vi "write_lockin_FP_DSC.vi"(8 "error in (no error)":errorcluster, 11 "front panel":T1 {"AI Configuration"."AI.Coupling" items=["AC"=10045, "DC"=10050, "GND"=10066]; "Channels: AO"."AO f (Hz)" min=0.001 max=10000.0; "Channels: AO"."AO DC (V)" format="%.3p"; "Channels: AO"."AO Amp (V)" format="%.3p"; "Channels: Lockin"."REF phi (°)" format="%#_3g"}) -> (0 "error out":errorcluster)   [LabVIEW 2016, in "Instrument.Lockin.lvclass"]
uses:
  Instrument.Lockin.lvclass
  Typedefs/Front Panel Cluster.ctl
  Typedefs/AO.config(UI)-array.ctl
  Typedefs/AO.config(UI)-cluster.ctl
  Typedefs/446xAO-enum.ctl
  Typedefs/AI.config(UI)-array.ctl
  Typedefs/AI.config(UI)-cluster.ctl
  Typedefs/AI.coupling-enum.ctl
  Typedefs/446xAI-enum.ctl
  Typedefs/AO-cluster.ctl
  Typedefs/AO_Amp-array.ctl
  Typedefs/AO_DC-array.ctl
  Typedefs/AO_f-array.ctl
  Typedefs/AO_phi-array.ctl
  Typedefs/Function-array.ctl
  Typedefs/Function-enum.ctl
  Typedefs/REF-cluster.ctl
  Typedefs/REF_f-array.ctl
  Typedefs/REF_phi-array.ctl
  Typedefs/DAQType-enum.ctl
  Typedefs/AmplifierType-enum.ctl
  Typedefs/Cal Info - Cluster.ctl
  <vilib>/Utility/sysdir.llb/System Directory Type.ctl
  <vilib>/addons/_JKI.lib/Serialization/JSON/JKI JSON Serialization.lvlib
panel:
  # "1"
  # "2"
  # "3"
  # "4"
  # "5"
  # "6"
  # "7"
  # "8"
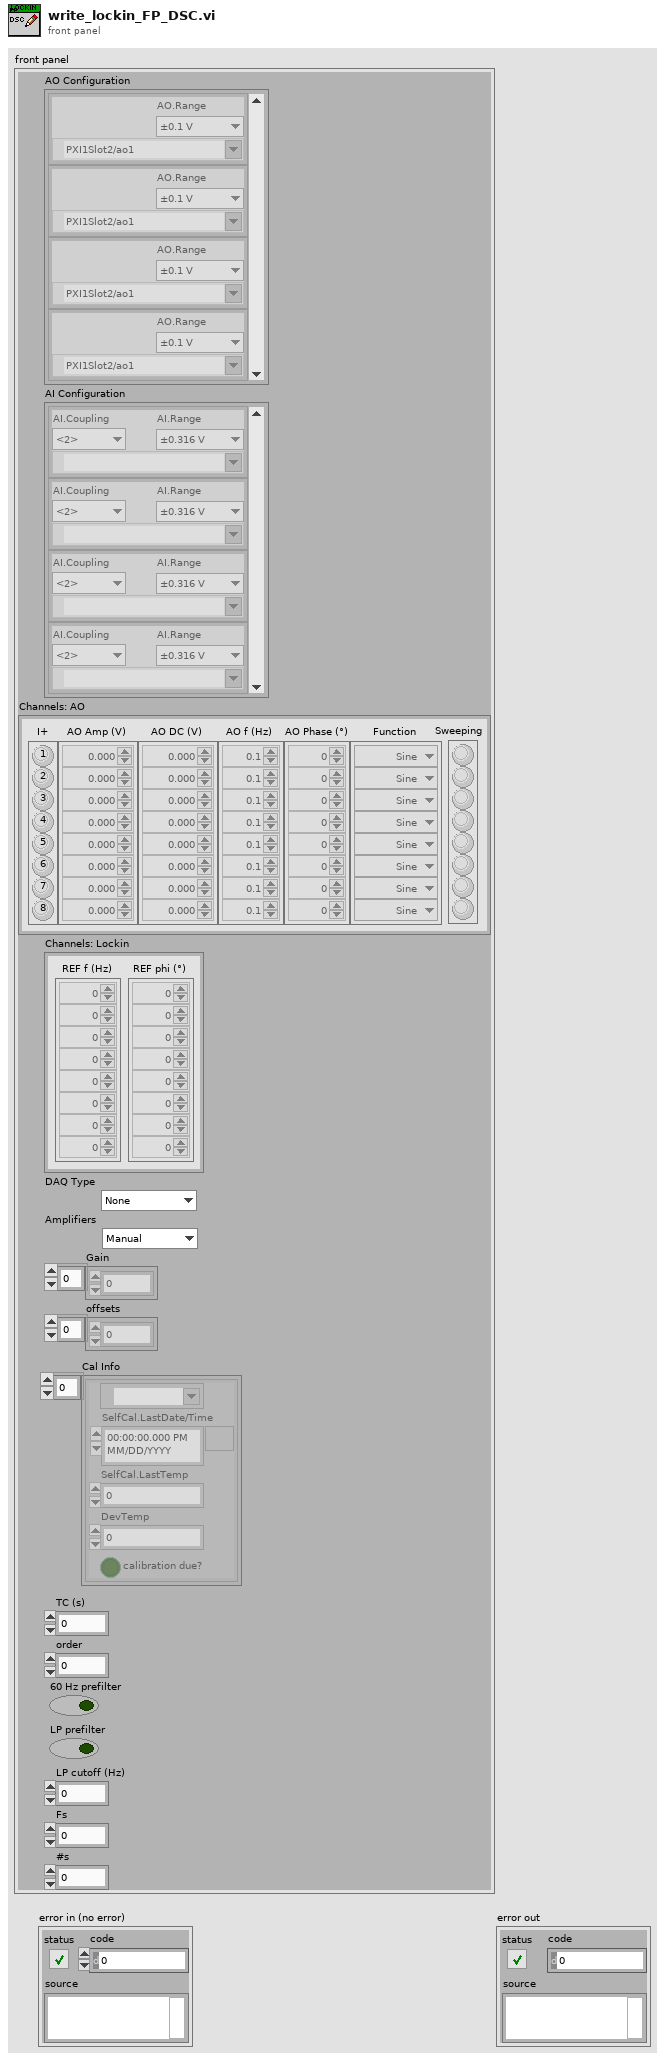
[diagram p1: front panel]
types:
  T1 = typedef "Instrument.Lockin.lvclass/Front Panel Cluster.ctl" = cluster{"AO Configuration":T2, "AI Configuration":T5, "Channels: AO":T9, "Channels: Lockin":T16, "DAQ Type":T19, "Amplifiers":T20, "Gain":dbl[], "offsets":dbl[], "Cal Info":T21[], "TC (s)":dbl, "order":i32, "60 Hz prefilter":bool, "LP prefilter":bool, "LP cutoff (Hz)":dbl, "Fs":i32, "#s":i32}
  T2 = typedef "Instrument.Lockin.lvclass/AO.config(UI)-array.ctl" = T3[]
  T3 = typedef "Instrument.Lockin.lvclass/AO.config(UI)-cluster.ctl" = cluster{"AO.Range":T4, "AO.channels":tag}
  T4 = typedef "Instrument.Lockin.lvclass/446xAO-enum.ctl" = enum16{"±0.1 V", "±1.0 V", "±10.0 V"}
  T5 = typedef "Instrument.Lockin.lvclass/AI.config(UI)-array.ctl" = T6[]
  T6 = typedef "Instrument.Lockin.lvclass/AI.config(UI)-cluster.ctl" = cluster{"AI.Coupling":T7, "AI.channels":tag, "AI.Range":T8}
  T7 = typedef "Instrument.Lockin.lvclass/AI.coupling-enum.ctl" = u16
  T8 = typedef "Instrument.Lockin.lvclass/446xAI-enum.ctl" = enum16{"±0.316 V", "±1.00 V", "±3.16 V", "±10.0 V", "±31.6 V", "±42.4 V"}
  T9 = typedef "Instrument.Lockin.lvclass/AO-cluster.ctl" = cluster{"AO Amp (V)":T10, "AO DC (V)":T11, "AO f (Hz)":T12, "AO Phase (°)":T13, "Function":T14, "I+":bool[], "Sweeping":bool[]}
  T10 = typedef "Instrument.Lockin.lvclass/AO_Amp-array.ctl" = dbl[]
  T11 = typedef "Instrument.Lockin.lvclass/AO_DC-array.ctl" = dbl[]
  T12 = typedef "Instrument.Lockin.lvclass/AO_f-array.ctl" = dbl[]
  T13 = typedef "Instrument.Lockin.lvclass/AO_phi-array.ctl" = dbl[]
  T14 = typedef "Instrument.Lockin.lvclass/Function-array.ctl" = T15[]
  T15 = typedef "Instrument.Lockin.lvclass/Function-enum.ctl" = enum16{"Sine", "Triangle", "Square", "Sawtooth"}
  T16 = typedef "Instrument.Lockin.lvclass/REF-cluster.ctl" = cluster{"REF f (Hz)":T17, "REF phi (°)":T18}
  T17 = typedef "Instrument.Lockin.lvclass/REF_f-array.ctl" = dbl[]
  T18 = typedef "Instrument.Lockin.lvclass/REF_phi-array.ctl" = dbl[]
  T19 = typedef "Instrument.Lockin.lvclass/DAQType-enum.ctl" = enum16{"None", "USB 4431", "PXI 446x"}
  T20 = typedef "Instrument.Lockin.lvclass/AmplifierType-enum.ctl" = enum16{"Manual", "Krohn Hite", "Femto"}
  T21 = typedef "Instrument.Lockin.lvclass/Cal Info - Cluster.ctl" = cluster{"Active Device":tag, "SelfCal.LastDate/Time":timestamp, "SelfCal.LastTemp":dbl, "DevTemp":dbl, "calibration due?":bool}
  T22 = typedef "System Directory Type.ctl" = i32
  T23 = cluster{"AO Configuration":cluster{"AO.Range":T4, "AO.channels":string}[], "AI Configuration":cluster{"AI.Coupling":T7, "AI.channels":string, "AI.Range":T8}[], "Channels: AO":T9, "Channels: Lockin":T16, "DAQ Type":T19, "Amplifiers":T20, "Gain":dbl[], "offsets":dbl[], "Cal Info":cluster{"Active Device":string, "SelfCal.LastDate/Time":timestamp, "SelfCal.LastTemp":dbl, "DevTemp":dbl, "calibration due?":bool}[], "TC (s)":dbl, "order":i32, "60 Hz prefilter":bool, "LP prefilter":bool, "LP cutoff (Hz)":dbl, "Fs":i32, "#s":i32}
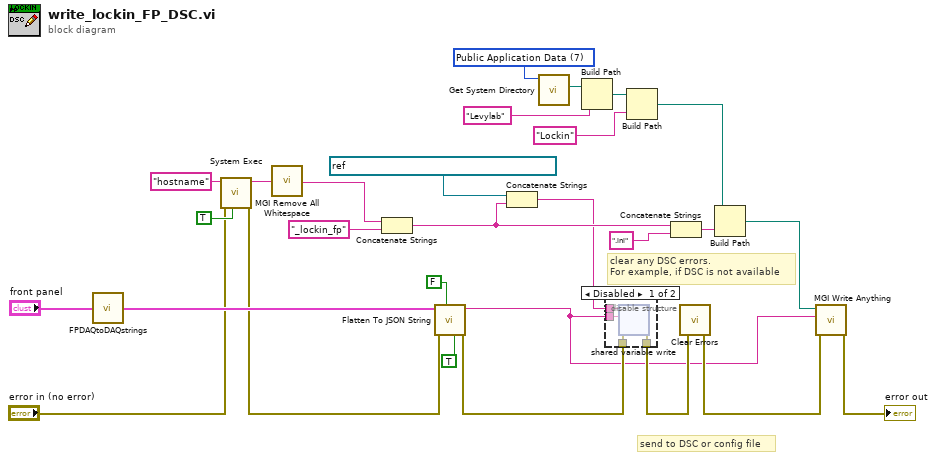
[diagram p0: block diagram]
diagram:
  w3 = T22 7 items=["User Home"=0, "User Desktop"=1, "User Documents"=2, "User Application Data"=3, "User Preferences"=4, "User Temporary"=5, "Public Documents"=6, "Public Application Data"=7, "Public Preferences"=8, "Public Cache"=13, "System Core Libraries"=9, "System Installed Libraries"=10, "Application Files"=11, "Boot Volume Root"=12] ("system directory type")
  # "clear any DSC errors.\nFor example, if DSC is not available"
  # "send to DSC or config file"
  n1 = call "FPDAQtoDAQstrings.vi"("front panel"="front panel") -> ("front panel (DAQmx strings)"=w23:T23)
  n2 = call <vilib>:"System Exec.vi"("run minimized? (F)"=TRUE, "error in (no error)"="error in (no error)", "command line"="hostname") -> ("error out"=w13:errorcluster, "standard output"=w16:string)  [unwired: 5 in, 2 out]
  n3 = call <userlib>:"MGI Remove All Whitespace.vi"("String"=w16) -> ("Trimmed String"=w11:string)
  n4 = Concatenate Strings(w11, "_lockin_fp" ("regular expression")) -> (w10:string)
  n5 = call <vilib>:"Flatten To JSON String.vi"("Enums As String (F)"=TRUE, "Multiline (T)"=FALSE, "error in (no error)"=w13, "Variant"=w23) -> ("error out"=w27:errorcluster, "JSON String"=w8:string)  [unwired: 6 in]
  n6 = Concatenate Strings(refnum<k21> "ni.var.psp://housesoftheholy/lockins/" ("shared variable refnum in"), w10) -> (w7:string)
  n7 = call <vilib>:"Get System Directory.vi"("system directory type"=w3) -> ("system directory"=w6:path)  [unwired: 10 in]
  n8 = Build Path(base path=w6, name or relative path="Levylab") -> (appended path=w4:path)
  n9 = disable-structure shown="Disabled" {
    disable-tunnel: w27 -> [w32 _]
    disable-tunnel: [w31 _] -> w22
    disable-tunnel: w8 -> [w30 _]
    disable-tunnel: w7 -> [w29 _]
    frame Disabled {
      n10 = shared-variable-write(w29, w32, w30) -> (w31:errorcluster)  [unwired: 1 out]
    }
    frame Enabled {
    }
  }
  n11 = Build Path(base path=w4, name or relative path="Lockin") -> (appended path=w1:path)
  n12 = Concatenate Strings(w10, ".ini" ("name or relative path")) -> (w19:string)
  n13 = call <vilib>:"Clear Errors.vi"("error in (no error)"=w22) -> ("error out"=w15:errorcluster)  [unwired: 5 in, 1 out]
  n14 = Build Path(base path=w1, name or relative path=w19) -> (appended path=w21:path)
  n15 = call <userlib>:"MGI Write Anything.vi"("Error In"=w15, "Anything"=w8, "Path (dialog)"=w21) -> ("Error Out"=→"error out":errorcluster)  [unwired: 6 in, 2 out]
